vi "Configure Average.vi"(8 "error in (no error)":errorcluster, 10 "Enable Statistics (F: Disable)":bool, 11 "VISA resource name":refnum<visa-resource-name>) -> (0 "error out":errorcluster, 3 "VISA resource name out":refnum<visa-resource-name>)   [LabVIEW 2020, in "Agilent 3446X Series.lvlib"]
doc: "Enables or disables statistics computation."
uses:
  Agilent 3446X Series.lvlib
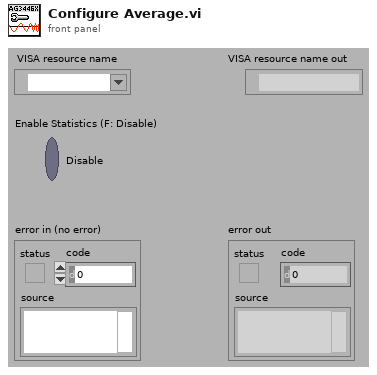
[diagram p1: front panel]
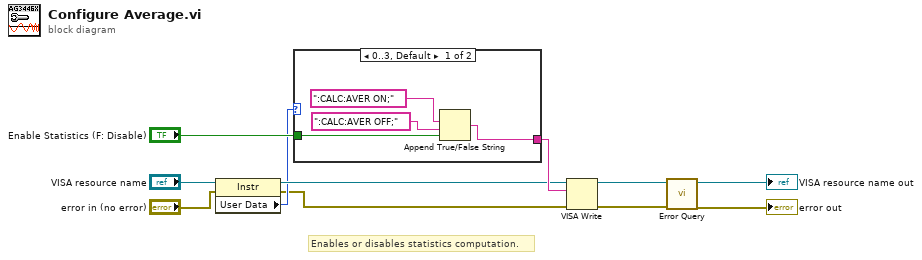
[diagram p0: block diagram]
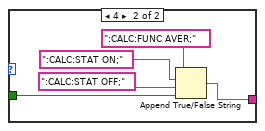
[diagram p2: hidden frame]
diagram:
  # "Enables or disables statistics computation."
  n1 = property class="Instr"(reference="VISA resource name", error in="error in (no error)") -> (reference out=w4:refnum<visa-resource-name>, error out=w1:errorcluster, "User Data"=w3:u32)
  n2 = case shown="0..3, Default" w3 {
    tunnel: "Enable Statistics (F: Disable)" -> [w15 w16]
    tunnel: [w12 w19] -> w10
    frame 0..3, Default {
      n3 = Append True/False String(1:w15, 2:":CALC:AVER OFF;", 3:":CALC:AVER ON;") -> (0:w12:string)  [unwired: 1 out]
    }
    frame 4 {
      n4 = Append True/False String(1:w16, 2:":CALC:STAT OFF;", 3:":CALC:STAT ON;", 4:":CALC:FUNC AVER;") -> (0:w19:string)
    }
  }
  n5 = VISA Write(VISA resource name=w4, write buffer=w10, error in (no error)=w1) -> (VISA resource name out=w9:refnum<visa-resource-name>, error out=w8:errorcluster)  [unwired: 1 out]
  n6 = call "Error Query.vi"("error in (no error)"=w8, "VISA resource name"=w9) -> ("error out"=→"error out":errorcluster, "VISA resource name out"=→"VISA resource name out":refnum<visa-resource-name>)  [unwired: 8 out]
